vi "poly_cast_boolean_notifier_n2q.vi"(2 "boolean notifier":T1) -> (7 "boolean queue":refnum<queue>)   [LabVIEW 2015]
uses:
  cores/boolean_notifier.ctl
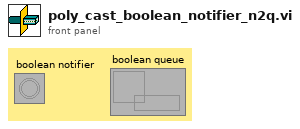
[diagram p1: front panel]
types:
  T1 = typedef "boolean_notifier.ctl" = refnum<k1>
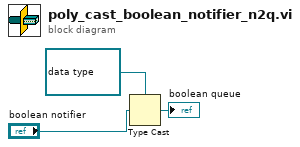
[diagram p0: block diagram]
diagram:
  n1 = Type Cast(type=refnum<queue> refnum ("boolean queue"), x="boolean notifier") -> (*(type *) &x=→"boolean queue":refnum<queue>)
